vi "ClientGUIMonitorAnalog.vi"() -> ()   [LabVIEW 2021]
doc: "Le protocole UDP diffère du protocole TCP car il n'y a pas de détection d'erreur avec les paquets d'informations qui sont envoyés ; il n'y a donc aucune garantie qu'un destinataire reçoive bien des données.\n\nLe protocole UDP offre la possibilité de diffuser des données sur un réseau. Spécifiez simplement une adresse IP de uns (255.255.255.255) pour essayer de diffuser l'information sur tout le réseau. Gardez à l'esprit que des routeurs et d'autres périphériques de réseau refusent généralement de diffuser au-delà de certains points, la diffusion est donc limitée dans la pratique."
panel:
  in  "Période\n(en ms)":u32(slide)=100 min=5 max=100 step=5 scale=5.0..100.0
  in  "Pin":u8=1 caption="Pin [0 - 11]" max=11
  out "Value":u16
  out "?":u16(graph)
  out "Response Command":u8[](array[numeric])
  in  "?":bool
  # "Version"
  # "Instruction"
  # "Argument[0]"
  # "Argument[1]"
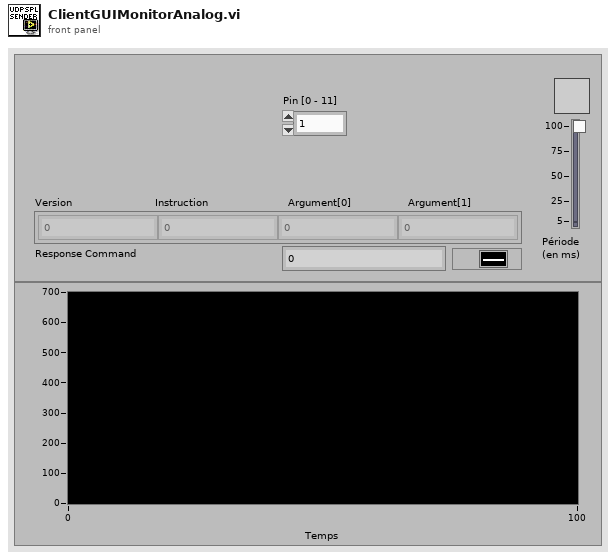
[diagram p1: front panel]
types:
  T1 = typedef "CommandType.ctl" = u8[]
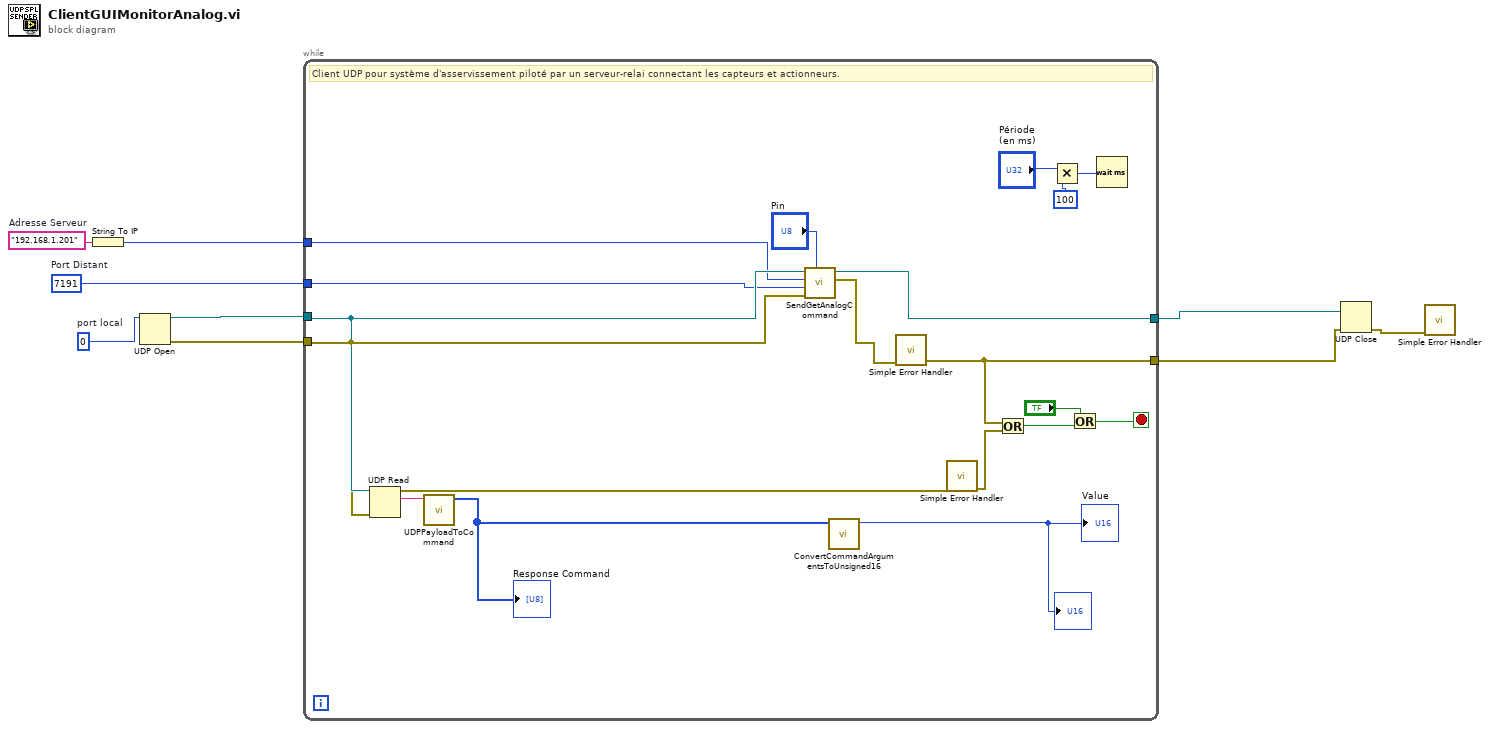
[diagram p0: block diagram]
diagram:
  w2 = u16 7191  # Port Distant
  w6 = u16 0  # port local
  w9 = "192.168.1.201"  # Adresse Serveur
  n1 = String To IP(1:w9) -> (0:w3:u32)
  n2 = UDP Open(11:w6) -> (port=w8:refnum<k16>, 0:w7:errorcluster)  [unwired: 4 in, 1 out]
  n3 = while {
    tunnel: w8 -> [w18]
    tunnel: w7 -> [w17]
    tunnel: [w16] -> w5
    tunnel: w3 -> [w14]
    tunnel: w2 -> [w13]
    tunnel: [w11] -> w1
    stop <- w25 stop-if-true
    # "Client UDP pour système d'asservissement piloté par un serveur-relai connectant les capteurs et actionneurs."
    n4 = UDP Read(connection ID=w18, 8:w17) -> (data out=w28:string, error out=w24:errorcluster)  [unwired: 2 in, 3 out]
    n5 = call "UDPPayloadToCommand.vi"("UDP Payload"=w28) -> ("Command"=w10:T1)  [unwired: 10 in]
    "Response Command" <- w10
    n6 = call "SendGetAnalogCommand.vi"("Pin"="Pin", "entrée d'erreur"=w17, "Port Destination"=w13, "Adresse IP Destination"=w14, "Connexion réseau UDP en entrée"=w18) -> ("sortie d'erreur 2"=w15:errorcluster, "Connexion réseau UDP en sortie"=w16:refnum<k16>)  [unwired: 5 in]
    n7 = call "ConvertCommandArgumentsToUnsigned16.vi"("Command"=w10) -> ("Numérique"=→"?" →"Value":u16)  [unwired: 10 in]
    n8 = call <vilib>:"Simple Error Handler.vi"("error in (no error)"=w15) -> ("error out"=w11:errorcluster)  [unwired: 4 in, 4 out]
    n9 = call <vilib>:"Simple Error Handler.vi"("error in (no error)"=w24) -> ("error out"=w23:errorcluster)  [unwired: 4 in, 4 out]
    n10 = Or(x=w11, y=w23) -> (x .or. y?=w27:bool)
    n11 = Multiply(x="Période\n(en ms)", y=u32 100) -> (x*y=w22:u32)
    n12 = Or(x="?", y=w27) -> (x .or. y?=w25:bool)
    n13 = Wait (ms)(milliseconds to wait=w22) -> ()  [unwired: 1 out]
  }
  n14 = UDP Close(connection ID=w5, 8:w1) -> (error out=w4:errorcluster)  [unwired: 1 out]
  n15 = call <vilib>:"Simple Error Handler.vi"("error in (no error)"=w4) -> ()  [unwired: 4 in, 5 out]
